vi "Parameter.vi"(9 "In":string, 10 "VIId":string, 11 "VariablesRef":T4) -> ()   [LabVIEW 2018, in "TDKDCSource.lvlib"]
uses:
  TDKDCSource.lvlib
  <userlib>/_OpenG.lib/dictionary/dictionary.llb/Dictionary Object RefNum__ogtk.ctl
  <userlib>/_OpenG.lib/dictionary/dictionary.llb/Dictionary Object RefNum - Enum__ogtk.ctl
  <vilib>/addons/_JKI.lib/Serialization/JSON/JKI JSON Serialization.lvlib
panel:
  in  "Tab Control":enum32{"Config", "控件"}(tab)
  in  "ArrayType":T1(tab)
  in  "Configuration":T2={"Language Selector"=enum."SCPI", "Baud Rate"=enum."9600", "Address"=6}
  in  "TDK直流电源端口":refnum<visa-resource-name>
  in  "Reset Device":bool
  in  "ID Query":bool
  in  "方法(Method)":T3(ring)
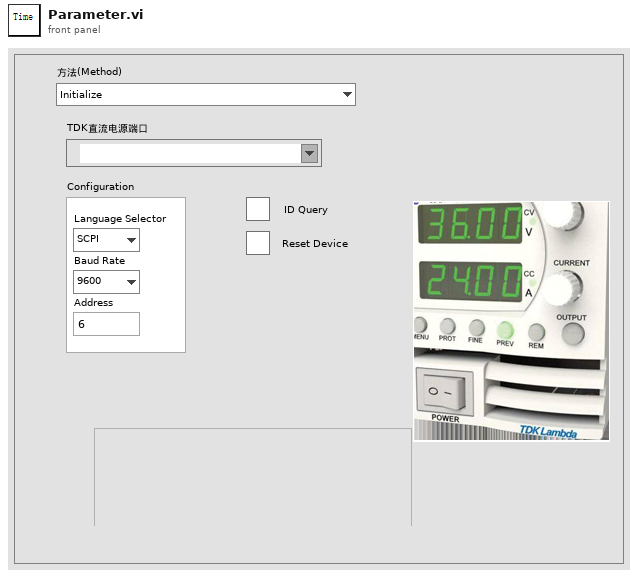
[diagram p1: front panel]
types:
  T1 = enum32{"Initialize", "SetVoltage", "SetCurrent", "SetOutput", "SetProtectedVoltage", "GetCurrent", "GetVoltage"}
  T2 = cluster{"Language Selector":enum16{"GEN", "SCPI"}, "Baud Rate":enum16{"1200", "2400", "4800", "9600", "19200", "38400", "57600", "115200"}, "Address":i16}
  T3 = enum16{"Initialize", "SetVoltage", "SetCurrent", "SetOutput", "SetProtectedVoltage", "GetCurrent", "GetVoltage", "GetPower"}
  T4 = typedef "Dictionary Object RefNum__ogtk.ctl" = refnum<k1>
  T5 = cluster{"Initialize":cluster{"json":cluster{"Method":string, "Time":i32, "ID Query":bool, "Reset Device":bool}}, "SetVoltage":cluster{"json":cluster{"Method":string, "Time":i32}}, "SetCurrent":cluster{"json":cluster{"Method":string}}}
  T6 = enum32{"Invalid", "Standard", "Closed", "Hidden", "Minimized", "Maximized"}
  T7 = enum32{"invalid app kind", "Development System", "Run Time System", "Student Edition", "Embedded LabVIEW", "Evaluation", "Custom"}
  T8 = cluster{"Core":cluster{"Current VI Reference":refnum<vi>, "Close Panel on Exit?":bool}, "Parameter":cluster{"VariableRef":T4}, "Synchronize":cluster{"EnqueueData":cluster{"Action":enum16{"Create", "Query", "Revert", "UpdateVariable", "Close"}, "Data":variant}, "Echo":cluster{"VIRef":refnum<vi>, "JsonOut":string, "Status":string}, "Communicate":cluster{"ID":string, "JsonIn":string, "VarRef":T4}, "Queue":refnum<queue>}, "TimeClusters":cluster{"Initialize":cluster{"json":cluster{"Method":string, "Time":i32, "ID Query":bool, "Reset Device":bool}}, "SetVoltage":cluster{"json":cluster{"Method":string, "Time":i32}}, "SetCurrent":cluster{"json":cluster{"Method":string}}}}
  T9 = cluster{"EnqueueData":cluster{"Action":enum16{"Create", "Query", "Revert", "UpdateVariable", "Close"}, "Data":variant}, "Echo":cluster{"VIRef":refnum<vi>, "JsonOut":string, "Status":string}, "Communicate":cluster{"ID":string, "JsonIn":string, "VarRef":T4}, "Queue":refnum<queue>}
  T10 = cluster{"Current VI Reference":refnum<vi>, "Close Panel on Exit?":bool}
  T11 = cluster{"json":cluster{"Method":string, "Time":i32, "ID Query":bool, "Reset Device":bool}}
  T12 = cluster{"json":cluster{"Method":string, "Time":i32}}
  T13 = cluster{"Action":enum16{"Create", "Query", "Revert", "UpdateVariable", "Close"}, "Data":variant}
  T14 = cluster{"ID":string, "JsonIn":string, "VarRef":T4}
  T15 = enum16{"Create", "Query", "Revert", "UpdateVariable", "Close"}
  T16 = cluster{"VIRef":refnum<vi>, "JsonOut":string, "Status":string}
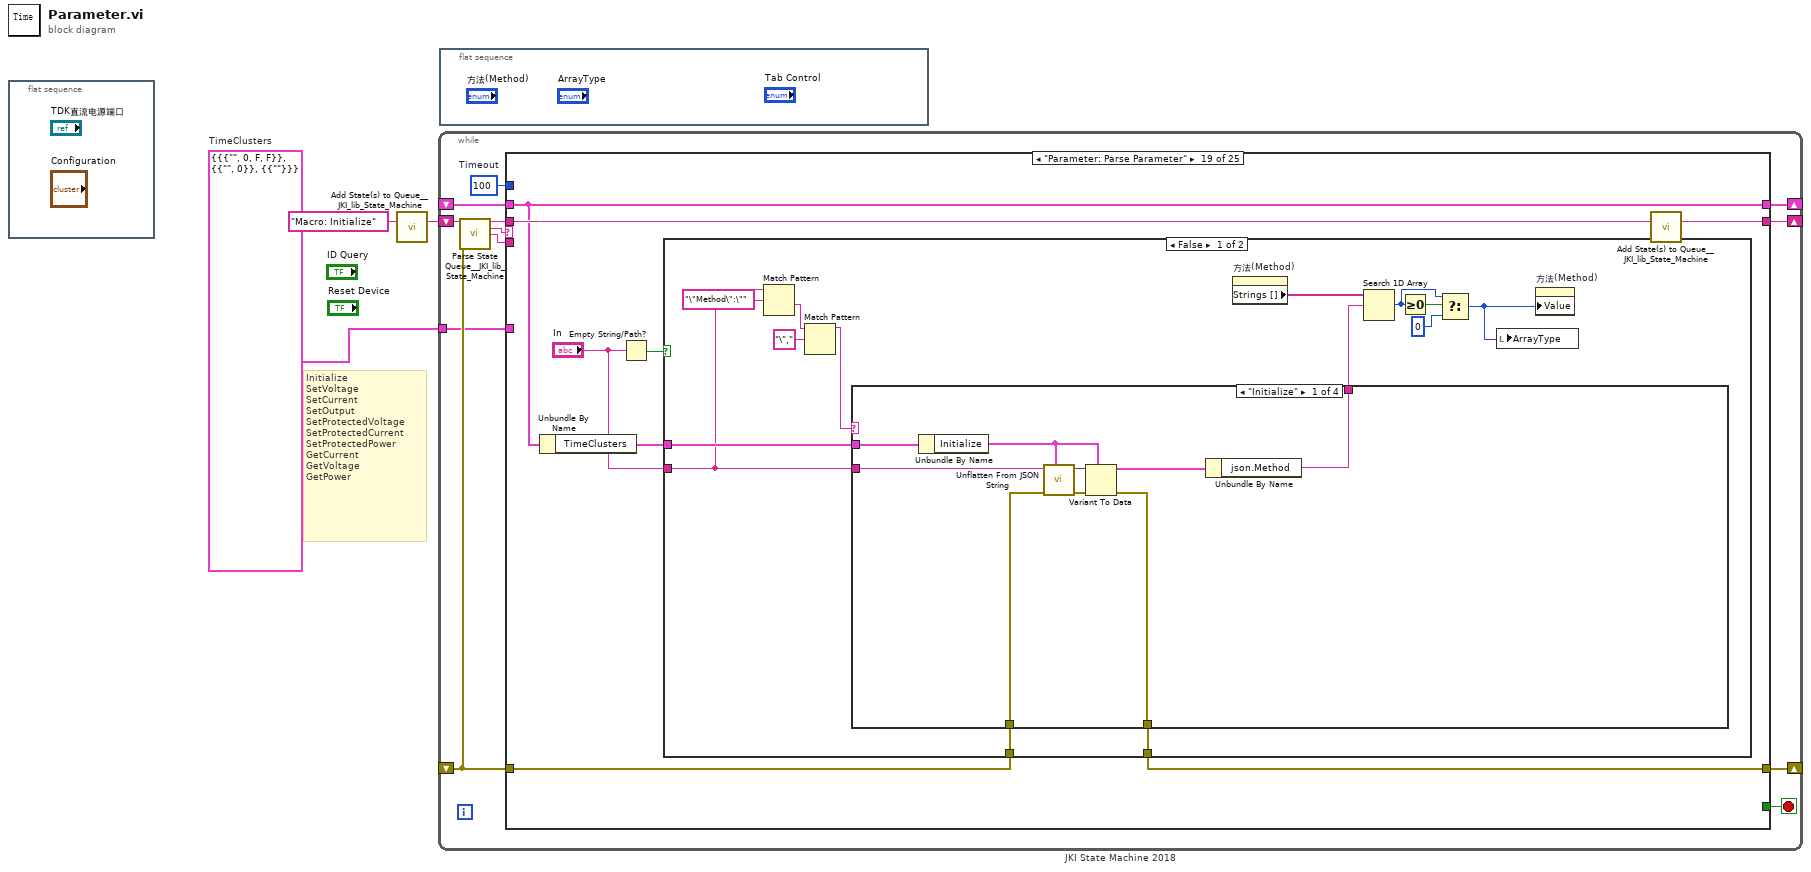
[diagram p0: block diagram]
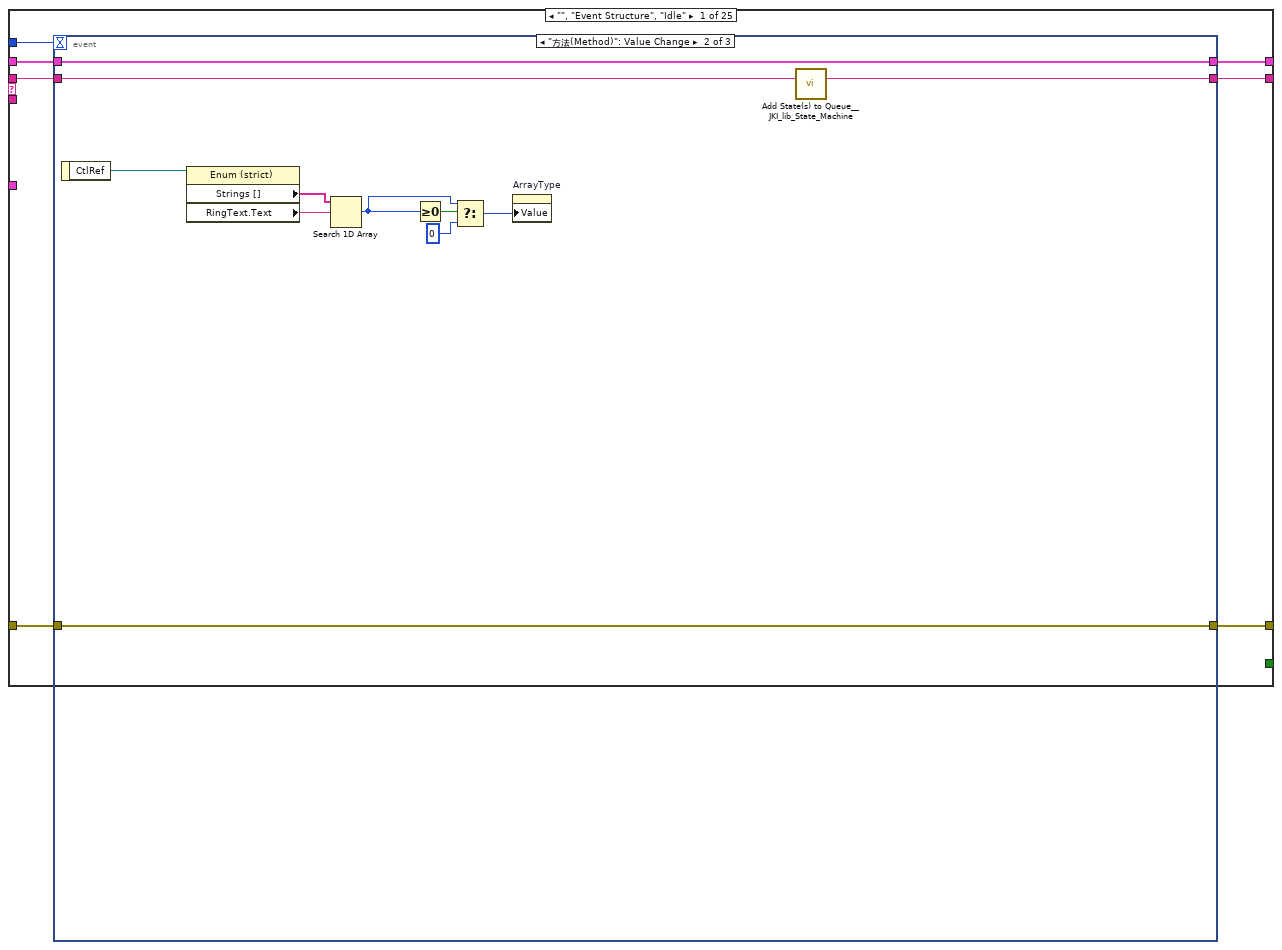
[diagram p2: hidden frame]
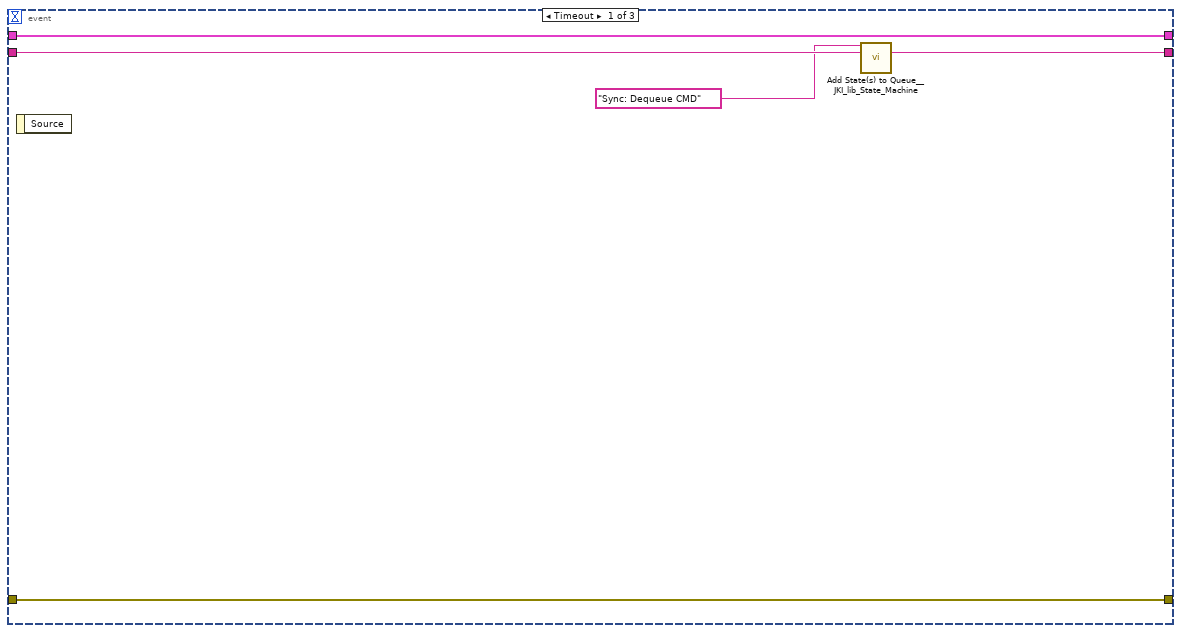
[diagram p3: hidden frame]
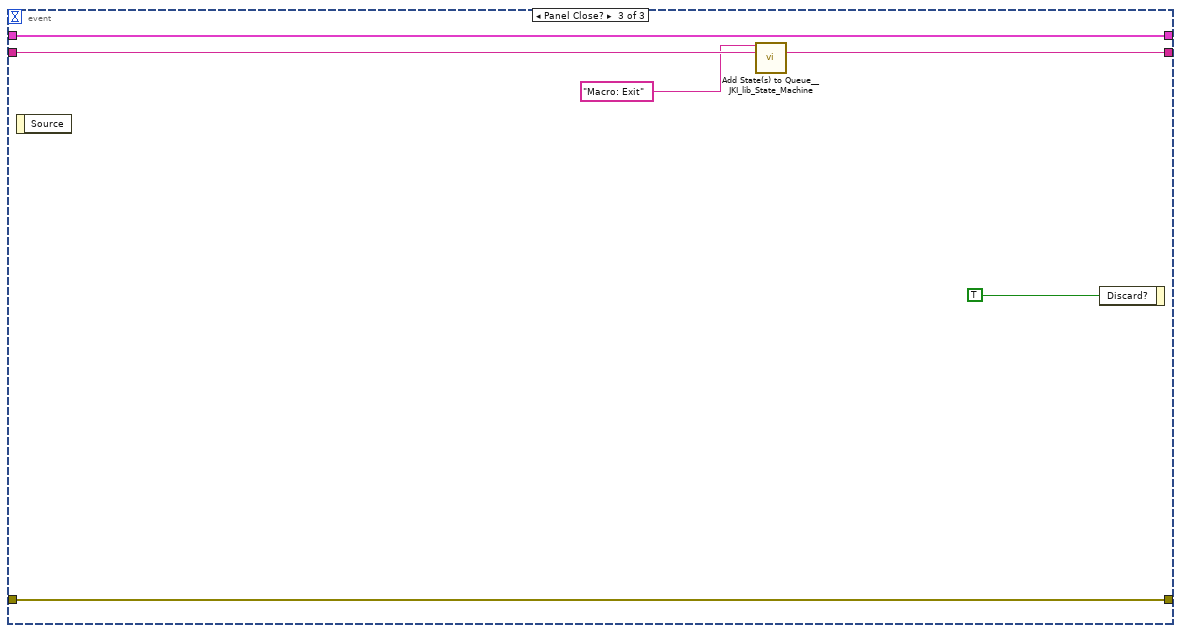
[diagram p4: hidden frame]
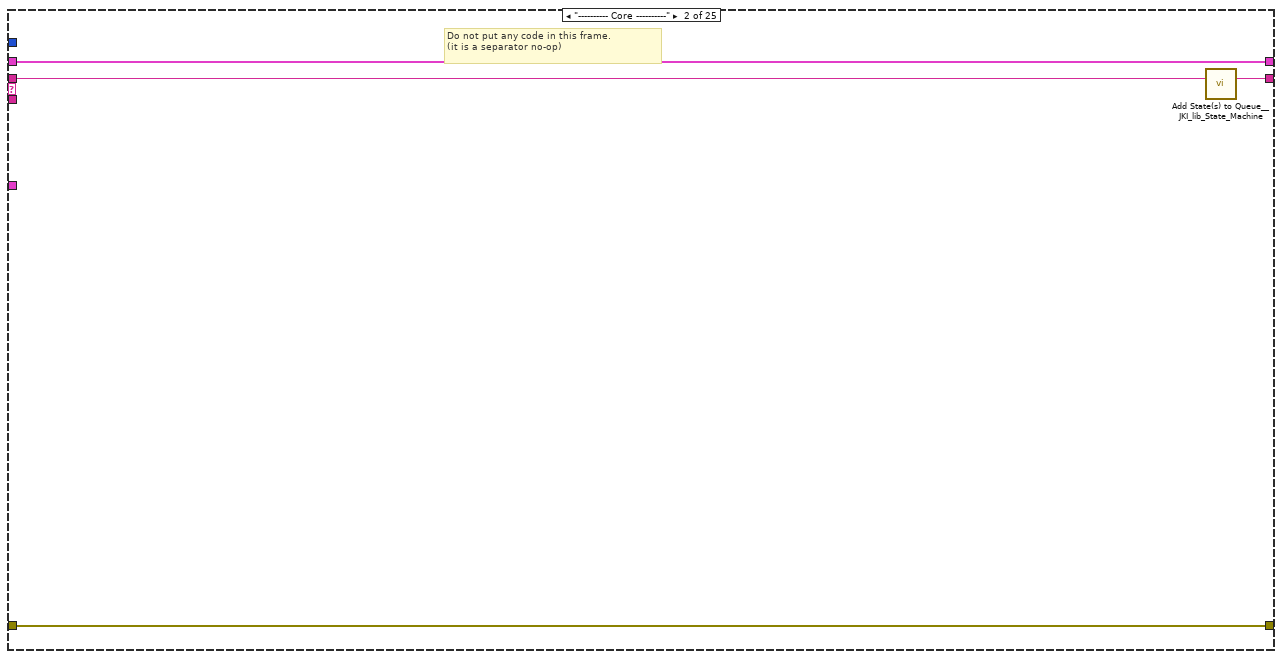
[diagram p5: hidden frame]
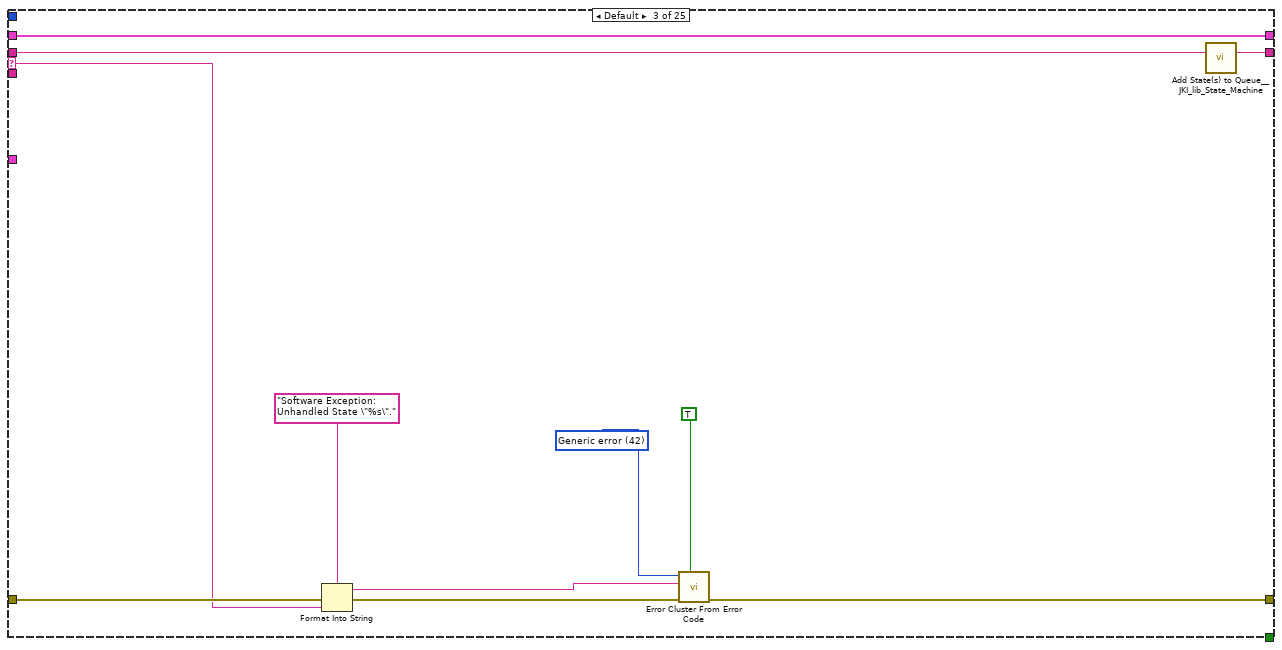
[diagram p6: hidden frame]
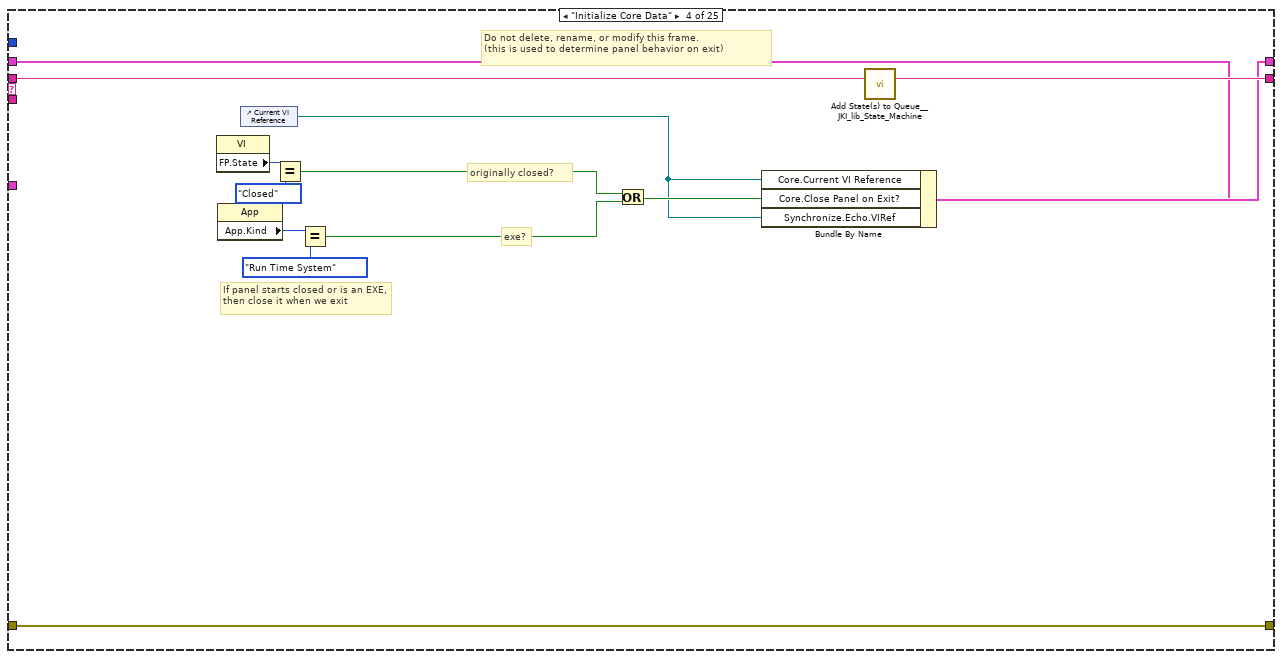
[diagram p7: hidden frame]
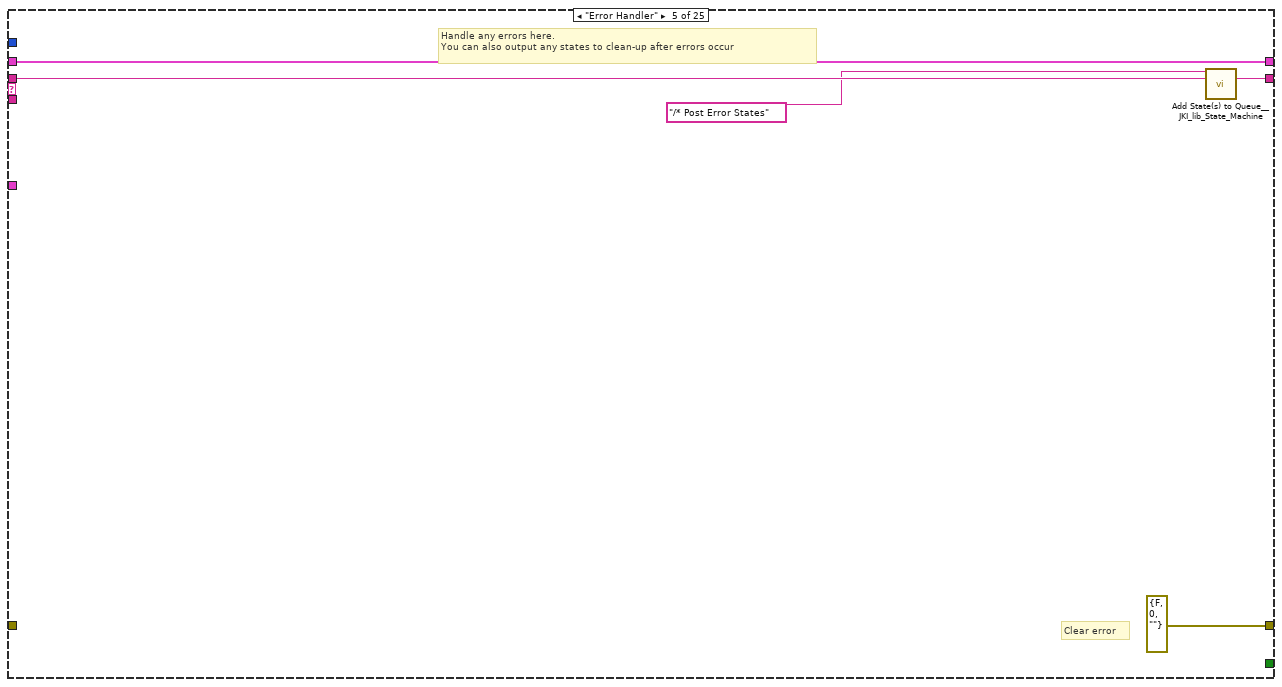
[diagram p8: hidden frame]
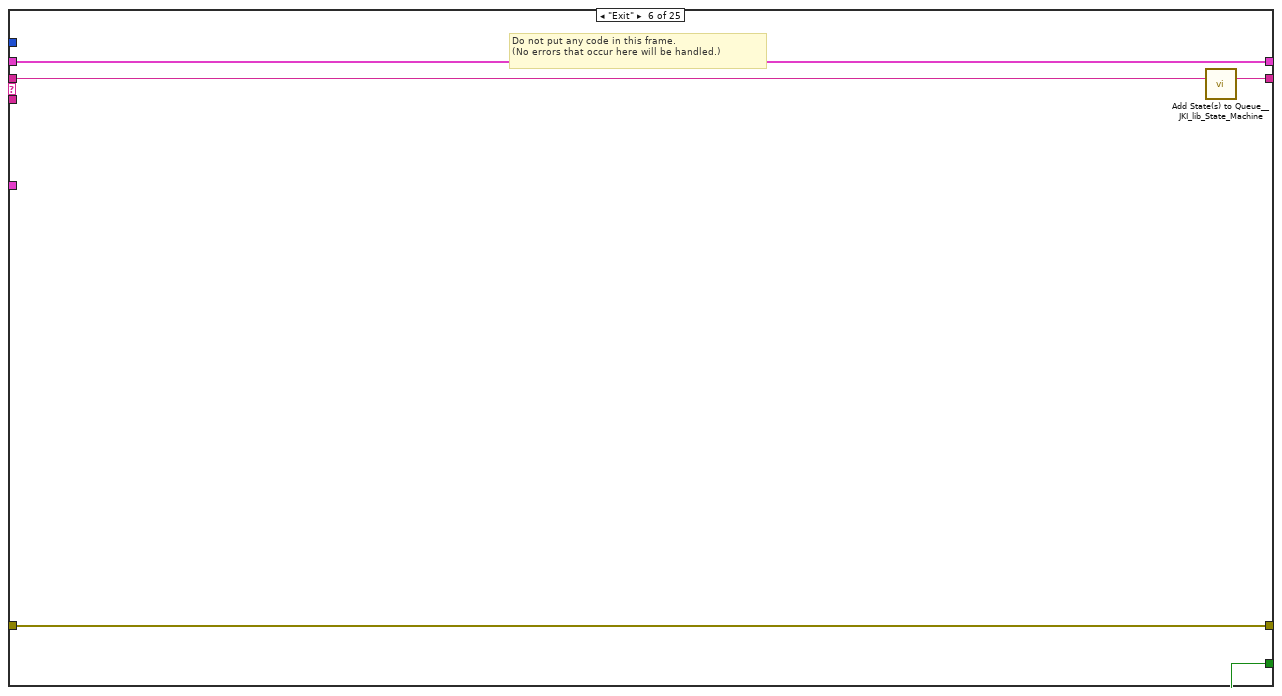
[diagram p9: hidden frame]
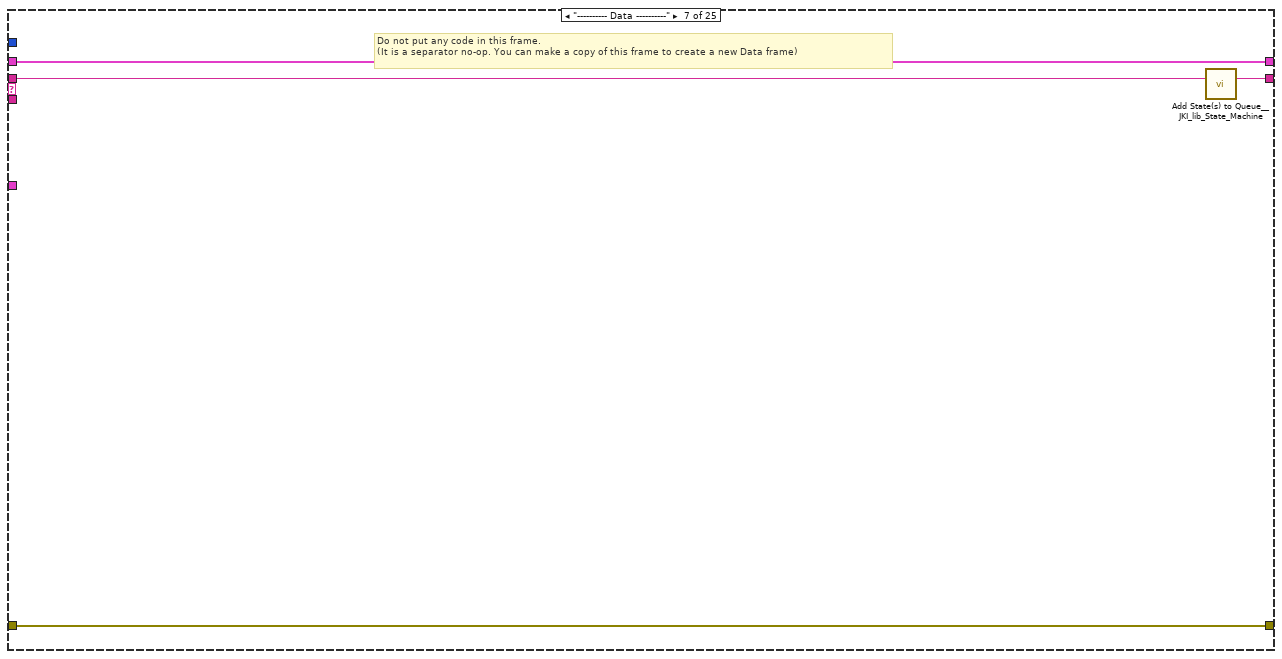
[diagram p10: hidden frame]
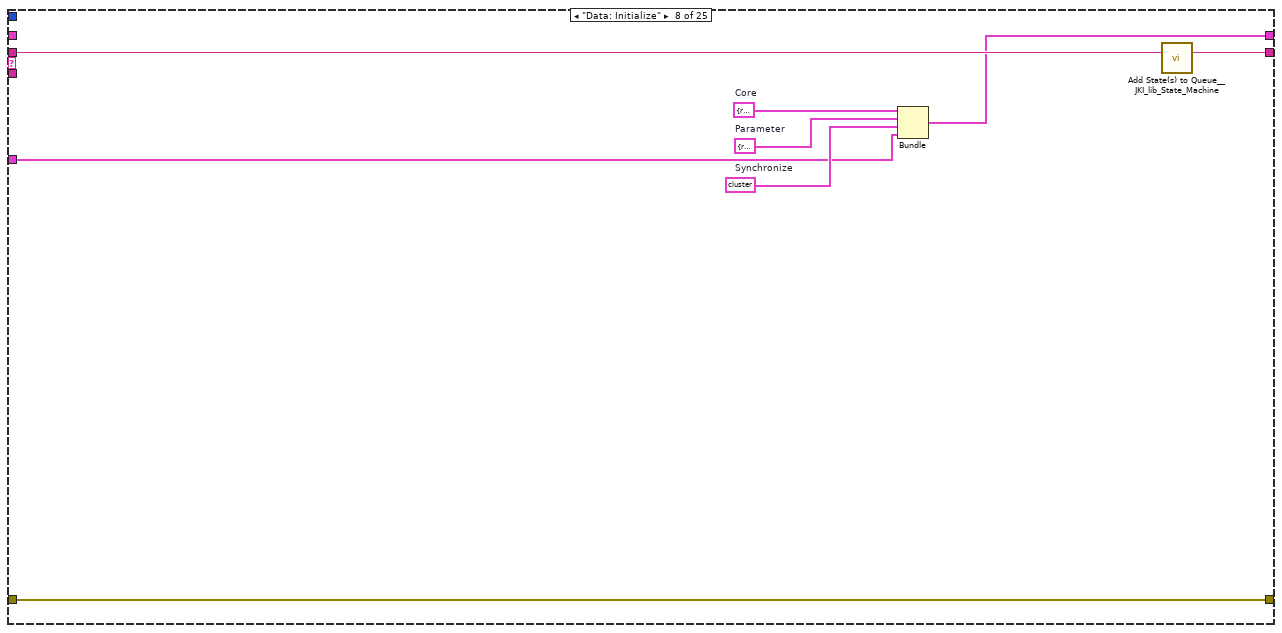
[diagram p11: hidden frame]
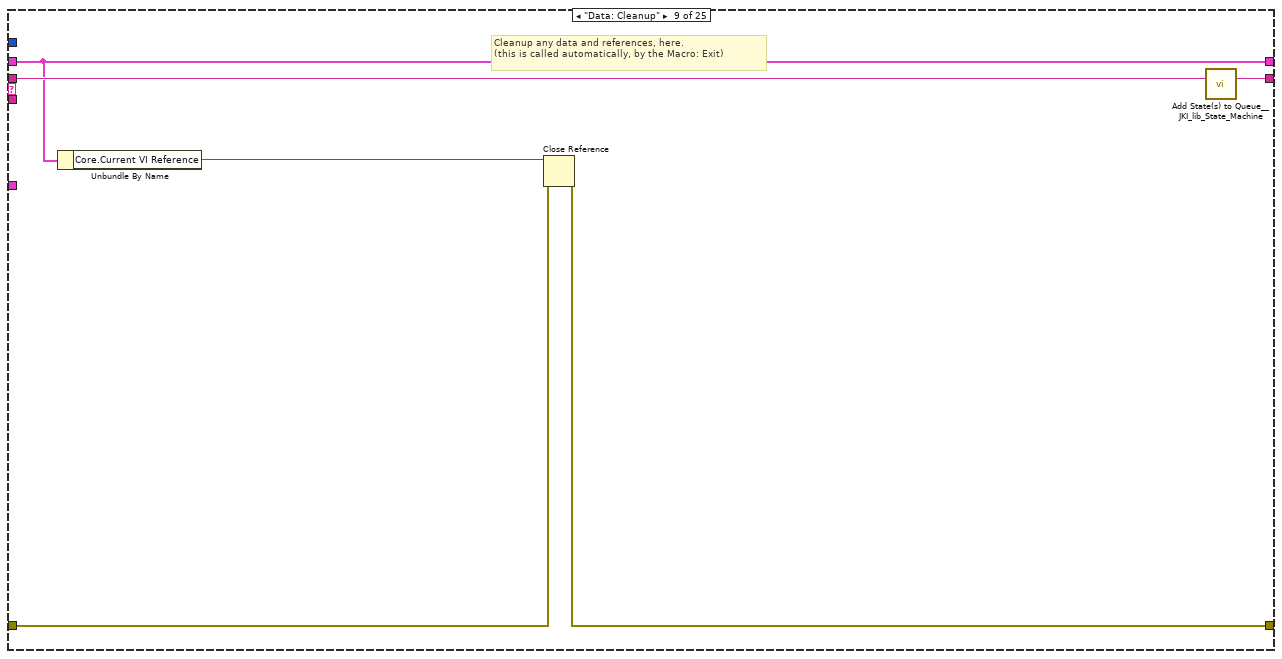
[diagram p12: hidden frame]
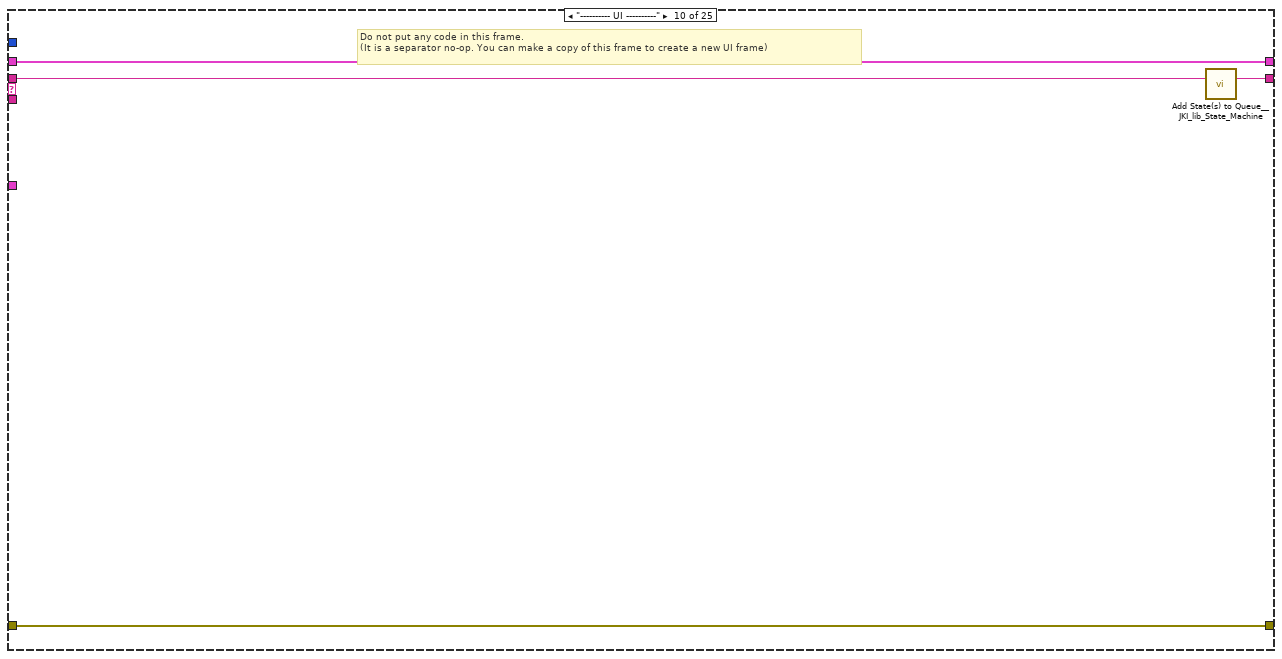
[diagram p13: hidden frame]
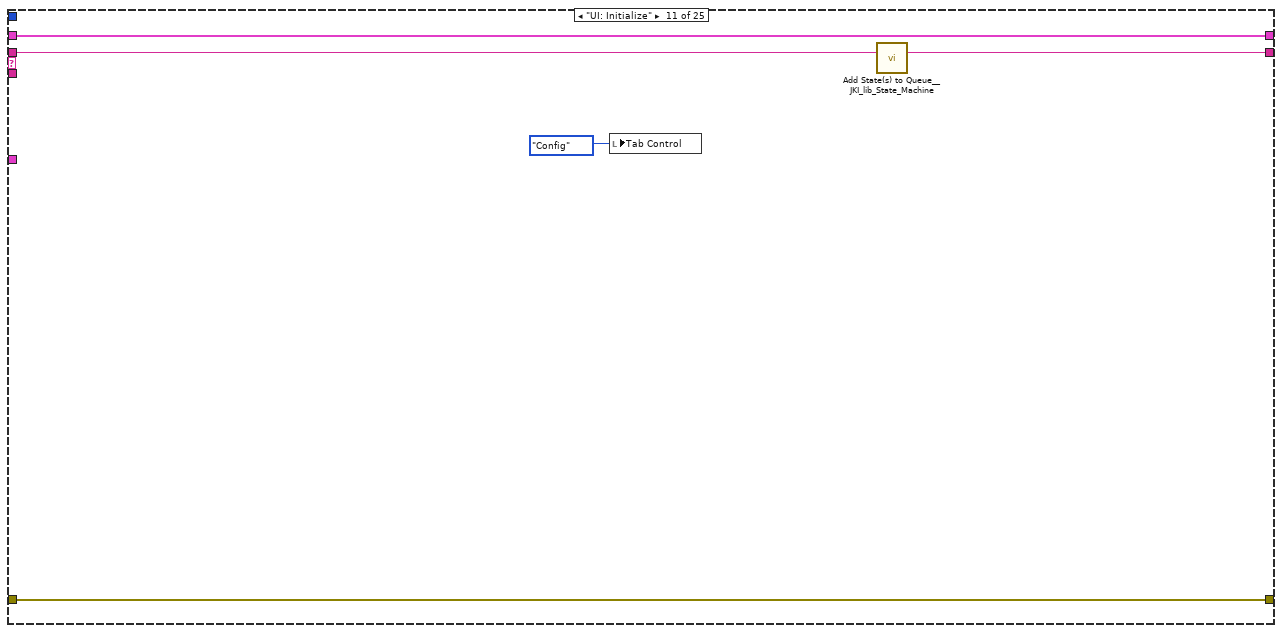
[diagram p14: hidden frame]
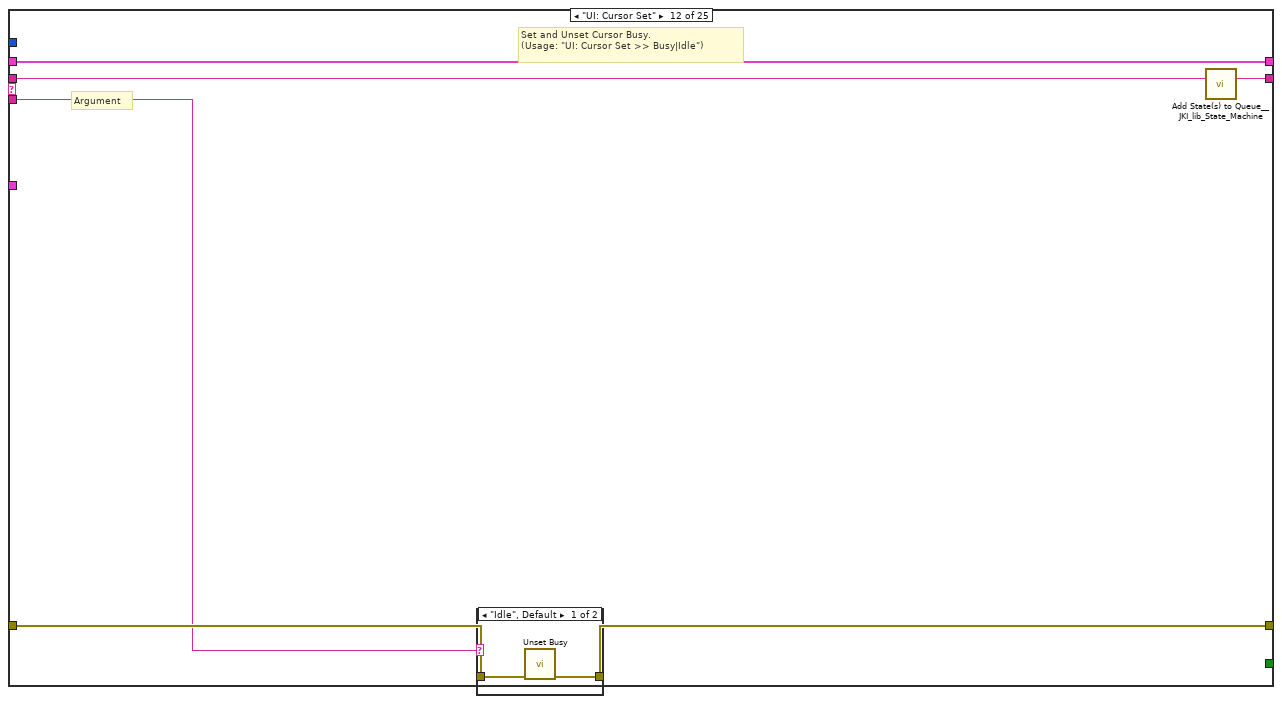
[diagram p15: hidden frame]
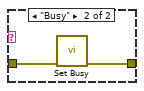
[diagram p16: hidden frame]
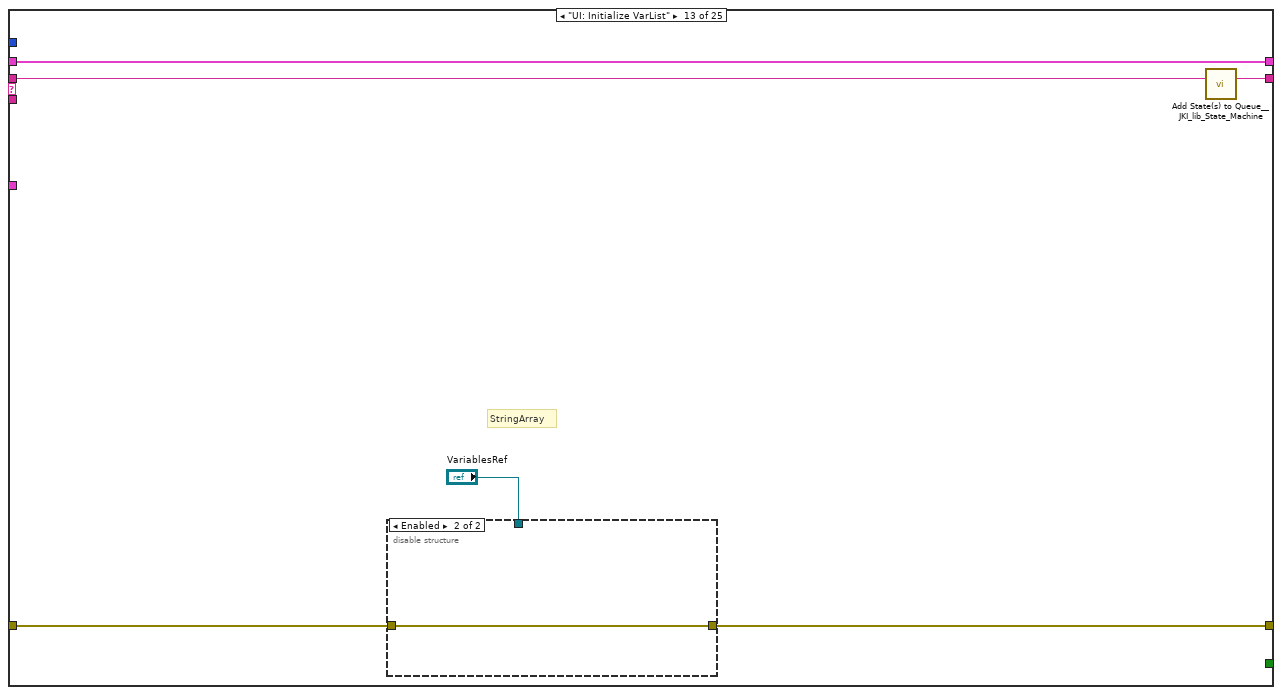
[diagram p17: hidden frame]
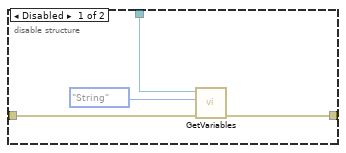
[diagram p18: hidden frame]
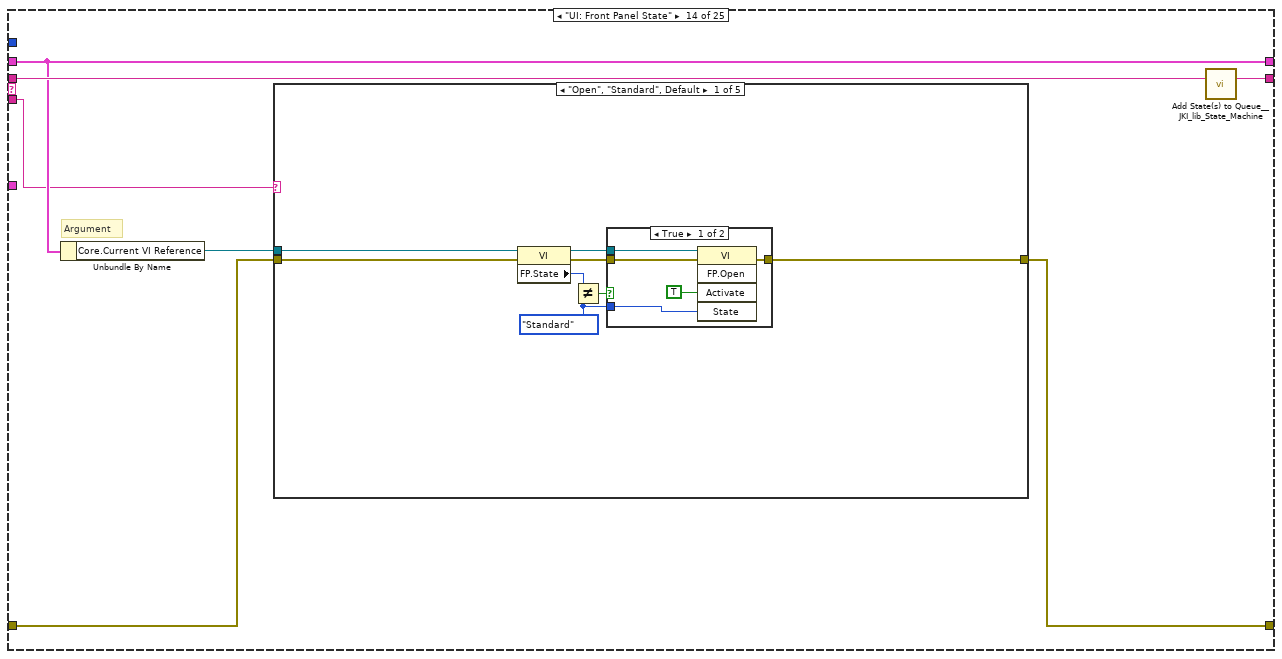
[diagram p19: hidden frame]
diagram:
  w1 = T5 {"Initialize"={"json"={"Method"="", "Time"=0, "ID Query"=FALSE, "Reset Device"=FALSE}}, "SetVoltage"={"json"={"Method"="", "Time"=0}}, "SetCurrent"={"json"={"Method"=""}}}  # TimeClusters
  # "Initialize\nSetVoltage\nSetCurrent\nSetOutput\nSetProtectedVoltage\nSetProtectedCurrent\nSetProtectedPower\nGetCurrent\nGetVoltage\nGetPower"
  n1 = flat-sequence {
    frame #0 {
    }
  }
  n2 = call <vilib>:"Add State(s) to Queue__JKI_lib_State_Machine.vi"("State(s) in (\"\")"="Macro: Initialize") -> ("States Out"=w3:string)  [unwired: 14 in]
  n3 = while "JKI State Machine 2018" {
    shift-right: [w8] -> _
    shift-left: _ -> [w7]
    shift-right: [w11] -> _
    shift-left: _ -> [w5]
    shift-right: [w10] -> _
    shift-left: w3 -> [w12]
    tunnel: w1 -> [w4]
    stop <- w9 stop-if-true
    w6 = 100  # Timeout
    n4 = call <vilib>:"Parse State Queue__JKI_lib_State_Machine.vi"("State Queue"=w12, "Error In (no error)"=w5) -> ("Remaining States"=w14:string, "Current State"=w15:string, "Arguments"=w13:string)  [unwired: 11 in]
    n5 = case shown="\"Parameter: Parse Parameter\"" w15 {
      selector: w15 -> [_ _ w49 _ _ _ _ _ _ _ _ _ _ _ _ _ _ _ _ _ _ _ _ _ _]
      tunnel: w14 -> [w22 w48 w53 w72 w77 w82 w86 w94 w100 w104 w109 w115 w125 w137 w206 w211 w221 w225 w233 w285 w314 w323 w338 w382 w397]
      tunnel: w13 -> [_ _ _ _ _ _ _ _ _ _ _ w110 _ w131 _ _ _ _ _ _ _ _ _ _ _]
      tunnel: w7 -> [w20 w45 w51 w65 w74 w80 w83 _ w95 w101 w106 w113 w123 w133 w203 w208 w218 w222 w228 w278 w311 w316 w336 w379 w386]
      tunnel: [w19 w46 w55 w69 errorcluster {"status"=FALSE, "code"=0, "source"=""} ("error out") w79 w84 w92 w96 w102 w105 w111 w120 w134 w204 w209 w219 w223 w229 w282 w312 w320 w325 w377 w384] -> w11
      tunnel: w5 -> [w18 w46 w54 w69 _ w79 w84 w92 w97 w102 w105 w112 w121 w135 w204 w209 w219 w223 w230 w281 w312 w321 w334 w378 w385]
      tunnel: [w21 w47 w52 w71 w76 w81 w85 w93 w99 w103 w108 w114 w124 w136 w205 w210 w220 w224 w232 w284 w313 w322 w337 w381 w396] -> w10
      tunnel: [_ _ _ _ _ TRUE _ _ _ _ _ _ _ _ _ _ _ _ _ _ _ _ _ _ _] -> w9
      tunnel: [w17 w45 w51 w70 w74 w80 w83 w89 w95 w101 w106 w113 w123 w133 w203 w208 w218 w222 w228 w283 w311 w318 w327 w379 w386] -> w8
      tunnel: w6 -> [w16 _ _ _ _ _ _ _ _ _ _ _ _ _ _ _ _ _ _ _ _ _ _ _ _]
      tunnel: w4 -> [_ _ _ _ _ _ _ w87 _ _ _ _ _ _ _ _ _ _ _ _ _ _ _ _ _]
      frame "", "Event Structure", "Idle" {
        n6 = event shown="[1] \"方法(Method)\": Value Change" {
          selector: _ -> [_ _ _]
          dyn-events: _ -> [_ _ _]
          timeout: w16 -> [_ _ _]
          tunnel: w22 -> [w27 w38 w44]
          tunnel: [w26 w37 w43] -> w21
          tunnel: w20 -> [w24 w35 w41]
          tunnel: [w25 w36 w42] -> w19
          tunnel: w18 -> [w25 w36 w42]
          tunnel: [w24 w35 w41] -> w17
          event Timeout {
            n7 = event-data() -> ()  [unwired: 1 in, 1 out]
            n8 = call <vilib>:"Add State(s) to Queue__JKI_lib_State_Machine.vi"("State(s) in Front (\"\")"="Sync: Dequeue CMD" ("State(s) in Front (\"\")"), "State(s) in (\"\")"=w27) -> ("States Out"=w26:string)  [unwired: 13 in]
          }
          event "方法(Method)": Value Change {
            n9 = event-data() -> ("CtlRef"=w31:refnum<vi>)  [unwired: 1 in]
            n10 = property class="Enum (strict)"(reference=w31) -> ("Strings []"=w30:string[], "RingText.Text"=w29:string)  [unwired: 1 in, 2 out]
            n11 = Search 1D Array(1D array=w30, element=w29) -> (index of element=w33:i32)  [unwired: 1 in]
            n12 = Greater Or Equal To 0?(x=w33) -> (x >= 0?=w34:bool)
            n13 = Select(t=w33, s=w34, f=0) -> (s? t:f=w28:i32)
            n14 = property on="ArrayType" class="TabCtl (strict)"("Value"=w28) -> ()  [unwired: 2 in, 2 out]
            n15 = call <vilib>:"Add State(s) to Queue__JKI_lib_State_Machine.vi"("State(s) in (\"\")"=w38) -> ("States Out"=w37:string)  [unwired: 14 in]
          }
          event Panel Close? {
            n16 = event-data() -> ()  [unwired: 1 in, 1 out]
            n17 = call <vilib>:"Add State(s) to Queue__JKI_lib_State_Machine.vi"("State(s) in Front (\"\")"="Macro: Exit", "State(s) in (\"\")"=w44) -> ("States Out"=w43:string)  [unwired: 13 in]
            n18 = event-data("Discard?"=TRUE) -> ()  [unwired: 1 in, 1 out]
          }
        }
      }
      frame "---------- Core ----------" {
        # "Do not put any code in this frame.\n(it is a separator no-op)"
        n19 = call <vilib>:"Add State(s) to Queue__JKI_lib_State_Machine.vi"("State(s) in (\"\")"=w48) -> ("States Out"=w47:string)  [unwired: 14 in]
      }
      frame Default {
        w58 = 42 items=["No error", "Argument error", "Memory is full", "Out of zone", "End of file", "File already open", "Generic file I/O error", "File not found", "File permission error", "Disk is full", "Duplicate path", "Too many files open", "System feature not enabled", "Resource file not found", "Cannot add resource", "Resource not found", "Image not found", "Image memory error", "Pen does not exist", "Config type invalid", "Config token not found", "Config parse error", "Config memory error", "Bad external code format", "Bad external code offset", "External code not present", "Null window", "Destroy window error", "Null menu", "Print aborted", "Bad print record", "Print driver error", "Windows error during printing", "Memory error during printing", "Print dialog error", "Generic print error", "Invalid device refnum", "Device not found", "Device parameter error", "Device unit error", "Cannot open device", "Device call aborted", "Generic error", "Cancelled by user", "Object ID too low", "Object ID too high", "Object not in heap", "Unknown heap", "Unknown object (invalid DefProc)", "Unknown object (DefProc not in table)", "Message out of range", "Invalid (null) method", "Unknown message", "Manager call not supported", "Bad address", "Network operation in progress", "Network operation timed out", "Connection is busy", "Network attribute not supported", "Network error", "Address in use", "System out of memory", "Connection aborted", "Connection refused", "Not connected", "Already connected", "Connection closed", "Initialization error (interapplication manager)", "Bad occurrence", "Wait on unbound occurrence handler", "Occurrence queue overflow", "Datalog type conflict", "Unused", "Unrecognized type (interapplication manager)", "Memory corrupt", "Failed to make temporary DLL", "Old CIN version", "Drag socket not found", "Failed to load drop-object", "Failed to register OLE object", "Failed to release OLE object", "Format specifier type mismatch", "Unknown format specifier", "Too few format specifiers", "Too many format specifiers", "Scan failed", "Newer CIN version", "Error converting to variant", "Runtime menu error", "Password tampered", "Variant attribute not found", "Incompatible variant data type", "Event data is not available", "Event Store is not present", "Occurrence is not found", "Event Queue is not created", "Event info is not available", "Refnum passed is NULL", "Error retrieving Class GUID", "Error retrieving CoClass GUID", "Error retrieving TypeLib GUID.", "Bad built application magic bytes.", "Specific driver is different from the specific driver associated with the Logical Name.", "There is no session opened to the class driver.", "Max Error", "MAX - Error with config objects", "MAX - Error loading configuration", "MAX - Group not supported"]
        n20 = Format Into String(format string="Software Exception: Unhandled State \"%s\"." ("message"), error in=w54, w49) -> (resulting string=w57:string, error out=w56:errorcluster)  [unwired: 1 in]
        n21 = call <vilib>:"Error Cluster From Error Code.vi"("show call chain? (False)"=TRUE, "error in (no error)"=w56, "error message (\"\")"=w57, "error code (0)"=w58) -> ("error out"=w55:errorcluster)  [unwired: 5 in]
        n22 = call <vilib>:"Add State(s) to Queue__JKI_lib_State_Machine.vi"("State(s) in (\"\")"=w53) -> ("States Out"=w52:string)  [unwired: 14 in]
      }
      frame "Initialize Core Data" {
        # "Do not delete, rename, or modify this frame.\n(this is used to determine panel behavior on exit)"
        # "originally closed?"
        # "exe?"
        # "If panel starts closed or is an EXE, then close it when we exit"
        n23 = property class="VI"() -> ("FP.State"=w63:T6)  [unwired: 2 in, 2 out]
        n24 = property class="App"() -> ("App.Kind"=w68:T7)  [unwired: 2 in, 2 out]
        n25 = control-ref of="Current VI Reference"() -> (w60:refnum<vi>)
        n26 = Equal?(x=w63, y=T6."Closed" ("Front Panel Window:State")) -> (x = y?=w61:bool)
        n27 = Equal?(x=w68, y=T7."Run Time System" ("Application:Kind")) -> (x = y?=w66:bool)
        n28 = Or(x=w61, y=w66) -> (x .or. y?=w64:bool)
        n29 = Bundle By Name(cluster=w65, "Core.Current VI Reference"=w60, "Core.Close Panel on Exit?"=w64, "Synchronize.Echo.VIRef"=w60) -> (w70:T8)
        n30 = call <vilib>:"Add State(s) to Queue__JKI_lib_State_Machine.vi"("State(s) in (\"\")"=w72) -> ("States Out"=w71:string)  [unwired: 14 in]
      }
      frame "Error Handler" {
        # "Handle any errors here.\nYou can also output any states to clean-up after errors occur"
        # "Clear error"
        n31 = call <vilib>:"Add State(s) to Queue__JKI_lib_State_Machine.vi"("State(s) in Front (\"\")"="/* Post Error States", "State(s) in (\"\")"=w77) -> ("States Out"=w76:string)  [unwired: 13 in]
      }
      frame "Exit" {
        # "Do not put any code in this frame.\n(No errors that occur here will be handled.)"
        n32 = call <vilib>:"Add State(s) to Queue__JKI_lib_State_Machine.vi"("State(s) in (\"\")"=w82) -> ("States Out"=w81:string)  [unwired: 14 in]
      }
      frame "---------- Data ----------" {
        # "Do not put any code in this frame.\n(It is a separator no-op. You can make a copy of this frame to create a new Data frame)"
        n33 = call <vilib>:"Add State(s) to Queue__JKI_lib_State_Machine.vi"("State(s) in (\"\")"=w86) -> ("States Out"=w85:string)  [unwired: 14 in]
      }
      frame "Data: Initialize" {
        w88 = cluster{"VariableRef":T4} {"VariableRef"=refnum}  # Parameter
        w90 = T9 {"EnqueueData"={"Action"=enum."Create", "Data"=variant}, "Echo"={"VIRef"=refnum, "JsonOut"="", "Status"=""}, "Communicate"={"ID"="", "JsonIn"="", "VarRef"=refnum}, "Queue"=refnum}  # Synchronize
        w91 = T10 {"Current VI Reference"=refnum, "Close Panel on Exit?"=FALSE}  # Core
        n34 = Bundle("Core"=w91, "Parameter"=w88, "Synchronize"=w90, "TimeClusters"=w87) -> (w89:T8)  [unwired: 1 in]
        n35 = call <vilib>:"Add State(s) to Queue__JKI_lib_State_Machine.vi"("State(s) in (\"\")"=w94) -> ("States Out"=w93:string)  [unwired: 14 in]
      }
      frame "Data: Cleanup" {
        # "Cleanup any data and references, here.\n(this is called automatically, by the Macro: Exit)"
        n36 = Unbundle By Name(w95) -> ("Core.Current VI Reference"=w98:refnum<vi>)
        n37 = Close Reference(reference=w98, error in (no error)=w97) -> (error out=w96:errorcluster)
        n38 = call <vilib>:"Add State(s) to Queue__JKI_lib_State_Machine.vi"("State(s) in (\"\")"=w100) -> ("States Out"=w99:string)  [unwired: 14 in]
      }
      frame "---------- UI ----------" {
        # "Do not put any code in this frame.\n(It is a separator no-op. You can make a copy of this frame to create a new UI frame)"
        n39 = call <vilib>:"Add State(s) to Queue__JKI_lib_State_Machine.vi"("State(s) in (\"\")"=w104) -> ("States Out"=w103:string)  [unwired: 14 in]
      }
      frame "UI: Initialize" {
        n40 = local write "Tab Control"(enum32{"Config", "控件"}."Config" ("Tab Control")) -> ()
        n41 = call <vilib>:"Add State(s) to Queue__JKI_lib_State_Machine.vi"("State(s) in (\"\")"=w109) -> ("States Out"=w108:string)  [unwired: 14 in]
      }
      frame "UI: Cursor Set" {
        # "Argument"
        # "Set and Unset Cursor Busy.\n(Usage: \"UI: Cursor Set >> Busy|Idle\")"
        n42 = case shown="\"Idle\", Default" w110 {
          tunnel: w112 -> [w117 w119]
          tunnel: [w116 w118] -> w111
          frame "Idle", Default {
            n43 = call <vilib>:"Unset Busy.vi"("error in (no error)"=w117) -> ("error out"=w116:errorcluster)  [unwired: 10 in]
          }
          frame "Busy" {
            n44 = call <vilib>:"Set Busy.vi"("error in (no error)"=w119) -> ("error out"=w118:errorcluster)  [unwired: 9 in, 1 out]
          }
        }
        n45 = call <vilib>:"Add State(s) to Queue__JKI_lib_State_Machine.vi"("State(s) in (\"\")"=w115) -> ("States Out"=w114:string)  [unwired: 14 in]
      }
      frame "UI: Initialize VarList" {
        # "StringArray"
        n46 = disable-structure shown="Enabled" {
          disable-tunnel: "VariablesRef" -> [w129 _]
          disable-tunnel: w121 -> [w127 w130]
          disable-tunnel: [w126 w130] -> w120
          frame Disabled {
            n47 = call "GetVariables.vi"("error in (no error)"=w127, "VariableType"=enum16{"String", "StringArray"}."String", "DicRef"=w129) -> ("error out"=w126:errorcluster)  [unwired: 7 in, 1 out]
          }
          frame Enabled {
          }
        }
        n48 = call <vilib>:"Add State(s) to Queue__JKI_lib_State_Machine.vi"("State(s) in (\"\")"=w125) -> ("States Out"=w124:string)  [unwired: 14 in]
      }
      frame "UI: Front Panel State" {
        # "Argument"
        n49 = Unbundle By Name(w133) -> ("Core.Current VI Reference"=w132:refnum<vi>)
        n50 = case shown="\"Open\", \"Standard\", Default" w131 {
          tunnel: w135 -> [w143 w158 w169 w182 w195]
          tunnel: [w145 w159 w171 w184 w197] -> w134
          tunnel: w132 -> [w144 w156 w170 w183 w196]
          frame "Open", "Standard", Default {
            w138 = T6."Standard" ("State")
            n51 = property class="VI"(reference=w144, error in=w143) -> (reference out=w141:refnum<vi>, error out=w142:errorcluster, "FP.State"=w140:T6)
            n52 = Not Equal?(x=w140, y=w138) -> (x != y?=w139:bool)
            n53 = case shown="True" w139 {
              tunnel: [w149 w151] -> w145
              tunnel: w142 -> [w148 w151]
              tunnel: w141 -> [w147 _]
              tunnel: w138 -> [w146 _]
              frame True {
                n54 = invoke class="VI" method="FP.Open"(reference=w147, error in=w148, "Activate"=TRUE, "State"=w146) -> (error out=w149:errorcluster)  [unwired: 1 in, 4 out]
              }
              frame False {
              }
            }
          }
          frame "Close", "Closed" {
            n55 = property class="VI"(reference=w156, error in=w158) -> (reference out=w155:refnum<vi>, error out=w157:errorcluster, "FP.State"=w153:T6)
            n56 = Not Equal?(x=w153, y=T6."Closed" ("Front Panel Window:State")) -> (x != y?=w152:bool)
            n57 = case shown="True" w152 {
              tunnel: [w160 w163] -> w159
              tunnel: w157 -> [w160 w162]
              tunnel: w155 -> [_ w161]
              frame False {
              }
              frame True {
                n58 = invoke class="VI" method="FP.Close"(reference=w161, error in=w162) -> (error out=w163:errorcluster)  [unwired: 1 in, 2 out]
              }
            }
          }
          frame "Hidden", "Hide" {
            w164 = T6."Hidden" ("State")
            n59 = property class="VI"(reference=w170, error in=w169) -> (reference out=w167:refnum<vi>, error out=w168:errorcluster, "FP.State"=w166:T6)
            n60 = Not Equal?(x=w166, y=w164) -> (x != y?=w165:bool)
            n61 = case shown="True" w165 {
              tunnel: [w175 w176] -> w171
              tunnel: w168 -> [w174 w176]
              tunnel: w167 -> [w173 _]
              tunnel: w164 -> [w172 _]
              frame True {
                n62 = invoke class="VI" method="FP.Open"(reference=w173, error in=w174, "State"=w172) -> (error out=w175:errorcluster)  [unwired: 2 in, 4 out]
              }
              frame False {
              }
            }
          }
          frame "Minimize", "Minimized" {
            w177 = T6."Minimized" ("State")
            n63 = property class="VI"(reference=w183, error in=w182) -> (reference out=w180:refnum<vi>, error out=w181:errorcluster, "FP.State"=w179:T6)
            n64 = Not Equal?(x=w179, y=w177) -> (x != y?=w178:bool)
            n65 = case shown="True" w178 {
              tunnel: [w188 w189] -> w184
              tunnel: w181 -> [w187 w189]
              tunnel: w180 -> [w186 _]
              tunnel: w177 -> [w185 _]
              frame True {
                n66 = invoke class="VI" method="FP.Open"(reference=w186, error in=w187, "State"=w185) -> (error out=w188:errorcluster)  [unwired: 2 in, 4 out]
              }
              frame False {
              }
            }
          }
          frame "Maximize", "Maximized" {
            w190 = T6."Maximized" ("State")
            n67 = property class="VI"(reference=w196, error in=w195) -> (reference out=w193:refnum<vi>, error out=w194:errorcluster, "FP.State"=w192:T6)
            n68 = Not Equal?(x=w192, y=w190) -> (x != y?=w191:bool)
            n69 = case shown="True" w191 {
              tunnel: [w201 w202] -> w197
              tunnel: w194 -> [w200 w202]
              tunnel: w193 -> [w199 _]
              tunnel: w190 -> [w198 _]
              frame True {
                n70 = invoke class="VI" method="FP.Open"(reference=w199, error in=w200, "State"=w198) -> (error out=w201:errorcluster)  [unwired: 2 in, 4 out]
              }
              frame False {
              }
            }
          }
        }
        n71 = call <vilib>:"Add State(s) to Queue__JKI_lib_State_Machine.vi"("State(s) in (\"\")"=w137) -> ("States Out"=w136:string)  [unwired: 14 in]
      }
      frame "---------- Macro ----------" {
        n72 = call <vilib>:"Add State(s) to Queue__JKI_lib_State_Machine.vi"("State(s) in (\"\")"=w206) -> ("States Out"=w205:string)  [unwired: 14 in]
      }
      frame "Macro: Initialize" {
        n73 = call <vilib>:"Add State(s) to Queue__JKI_lib_State_Machine.vi"("State(s) in Front (\"\")"="Data: Initialize\nInitialize Core Data\nUI: Initialize\nSync: Obtain CMD Queue\nSync: Dequeue CMD\nUI: Initialize VarList\nParameter: Parse Parameter", "State(s) in (\"\")"=w211) -> ("States Out"=w210:string)  [unwired: 13 in]
      }
      frame "Macro: Exit" {
        n74 = Unbundle By Name(w218) -> ("Core.Close Panel on Exit?"=w217:bool)
        n75 = Select(t="UI: Front Panel State >> Close", s=w217, f="") -> (s? t:f=w214:string)
        n76 = call <vilib>:"Add State(s) to Queue__JKI_lib_State_Machine.vi"("State(s) in (\"\")"=w214, "State(s) at Back (\"\")"="Sync: Release CMD Queue\nData: Cleanup\nExit") -> ("States Out"=w212:string)  [unwired: 13 in]
        n77 = call <vilib>:"Add State(s) to Queue__JKI_lib_State_Machine.vi"("State(s) in Front (\"\")"=w212, "State(s) in (\"\")"=w221) -> ("States Out"=w220:string)  [unwired: 13 in]
      }
      frame "---------- Parameter ----------" {
        # "Template Separator\n(You can make a copy of, or modify, this frame)"
        n78 = call <vilib>:"Add State(s) to Queue__JKI_lib_State_Machine.vi"("State(s) in (\"\")"=w225) -> ("States Out"=w224:string)  [unwired: 14 in]
      }
      frame "Parameter: Parse Parameter" {
        n79 = Unbundle By Name(w228) -> ("TimeClusters"=w227:T5)
        n80 = Empty String/Path?(string/path="In") -> (empty?=w231:bool)
        n81 = case shown="False" w231 {
          tunnel: "In" -> [w242 _]
          tunnel: w230 -> [w247 w276]
          tunnel: [w246 w276] -> w229
          tunnel: w227 -> [w245 _]
          frame False {
            n82 = Match Pattern(string=w242, regular expression="\"Method\":\"") -> (after substring=w241:string)  [unwired: 1 in, 3 out]
            n83 = Match Pattern(string=w241, regular expression="\",") -> (before substring=w240:string)  [unwired: 1 in, 3 out]
            n84 = case shown="\"Initialize\"" w240 {
              tunnel: w242 -> [w254 w263 w272 _]
              tunnel: w247 -> [w252 w261 w270 w275]
              tunnel: [w251 w260 w269 w275] -> w246
              tunnel: w245 -> [w249 w258 w267 _]
              tunnel: [w250 w259 w268 _] -> w235
              frame "Initialize" {
                n85 = Unbundle By Name(w249) -> ("Initialize"=w248:T11)
                n86 = call <vilib>:"Unflatten From JSON String.vi"("Type and Defaults"=w248, "error in (no error)"=w252, "JSON String"=w254) -> ("error out"=w255:errorcluster, "Variant"=w256:variant)  [unwired: 7 in]
                n87 = Variant To Data(error in=w255, type=w248, Variant=w256) -> (data=w253:T11, error out=w251:errorcluster)
                n88 = Unbundle By Name(w253) -> ("json.Method"=w250:string)
              }
              frame "Wait_s" {
                n89 = Unbundle By Name(w258) -> ("SetVoltage"=w257:T12)
                n90 = call <vilib>:"Unflatten From JSON String.vi"("Type and Defaults"=w257, "error in (no error)"=w261, "JSON String"=w263) -> ("error out"=w264:errorcluster, "Variant"=w265:variant)  [unwired: 7 in]
                n91 = Variant To Data(error in=w264, type=w257, Variant=w265) -> (data=w262:T12, error out=w260:errorcluster)
                n92 = Unbundle By Name(w262) -> ("json.Method"=w259:string)  [unwired: 1 out]
              }
              frame "TickCount" {
                n93 = Unbundle By Name(w267) -> ("SetCurrent"=w266:cluster{"json":cluster{"Method":string}})
                n94 = call <vilib>:"Unflatten From JSON String.vi"("Type and Defaults"=w266, "error in (no error)"=w270, "JSON String"=w272) -> ("error out"=w273:errorcluster, "Variant"=w274:variant)  [unwired: 7 in]
                n95 = Variant To Data(error in=w273, type=w266, Variant=w274) -> (data=w271:cluster{"json":cluster{"Method":string}}, error out=w269:errorcluster)
                n96 = Unbundle By Name(w271) -> ("json.Method"=w268:string)
              }
              frame Default {
              }
            }
            n97 = property on="方法(Method)" class="Enum (strict)"() -> ("Strings []"=w237:string[])  [unwired: 2 in, 2 out]
            n98 = Search 1D Array(1D array=w237, element=w235) -> (index of element=w239:i32)  [unwired: 1 in]
            n99 = Greater Or Equal To 0?(x=w239) -> (x >= 0?=w238:bool)
            n100 = Select(t=w239, s=w238, f=0) -> (s? t:f=w234:i32)
            n101 = local write "ArrayType"(w234) -> ()
            n102 = property on="方法(Method)" class="Enum (strict)"("Value"=w234) -> ()  [unwired: 2 in, 2 out]
          }
          frame True {
          }
        }
        n103 = call <vilib>:"Add State(s) to Queue__JKI_lib_State_Machine.vi"("State(s) in (\"\")"=w233) -> ("States Out"=w232:string)  [unwired: 14 in]
      }
      frame "Parameter: Combin Parameter" {
        n104 = property on="方法(Method)" class="Enum (strict)"() -> ("RingText.Text"=w280:string)  [unwired: 2 in, 2 out]
        n105 = Unbundle By Name(w278) -> ("TimeClusters"=w277:T5)
        n106 = case shown="\"Wait_s\"" w280 {
          selector: w280 -> [_ w288 w296 w304]
          tunnel: w277 -> [_ w294 w302 w310]
          tunnel: [_ w292 w300 w308] -> w279
          tunnel: [w286 w287 w295 w303] -> w282
          tunnel: w281 -> [w286 w290 w298 w306]
          frame Default {
          }
          frame "Wait_ms" {
            n107 = Unbundle By Name(w294) -> ("Initialize"=w293:T11)
            n108 = Bundle By Name(cluster=w293, "json.Method"=w288) -> (w289:T11)
            n109 = call <vilib>:"Flatten To JSON String.vi"("Multiline (T)"=TRUE, "error in (no error)"=w290, "Variant"=w289) -> ("error out"=w287:errorcluster, "JSON String"=w292:string)  [unwired: 7 in]
          }
          frame "Wait_s" {
            n110 = Unbundle By Name(w302) -> ("SetVoltage"=w301:T12)
            n111 = Bundle By Name(cluster=w301, "json.Method"=w296) -> (w297:T12)
            n112 = call <vilib>:"Flatten To JSON String.vi"("Multiline (T)"=TRUE, "error in (no error)"=w298, "Variant"=w297) -> ("error out"=w295:errorcluster, "JSON String"=w300:string)  [unwired: 7 in]
          }
          frame "TickCount" {
            n113 = Unbundle By Name(w310) -> ("SetCurrent"=w309:cluster{"json":cluster{"Method":string}})
            n114 = Bundle By Name(cluster=w309, "json.Method"=w304) -> (w305:cluster{"json":cluster{"Method":string}})
            n115 = call <vilib>:"Flatten To JSON String.vi"("Multiline (T)"=TRUE, "error in (no error)"=w306, "Variant"=w305) -> ("error out"=w303:errorcluster, "JSON String"=w308:string)  [unwired: 7 in]
          }
        }
        n116 = Bundle By Name(cluster=w278, "Synchronize.Echo.JsonOut"=w279) -> (w283:T8)
        n117 = call <vilib>:"Add State(s) to Queue__JKI_lib_State_Machine.vi"("State(s) in (\"\")"=w285) -> ("States Out"=w284:string)  [unwired: 14 in]
      }
      frame "---------- Sync ----------" {
        n118 = call <vilib>:"Add State(s) to Queue__JKI_lib_State_Machine.vi"("State(s) in (\"\")"=w314) -> ("States Out"=w313:string)  [unwired: 14 in]
      }
      frame "Sync: Obtain CMD Queue" {
        # "这里由平台输入"
        n119 = Unbundle By Name(w316) -> ("Synchronize.EnqueueData"=w315:T13)
        n120 = Obtain Queue(name (unnamed)="VIId", element data type=w315, error in (no error)=w321) -> (queue out=w317:refnum<queue>, error out=w320:errorcluster)  [unwired: 2 in, 1 out]
        n121 = Bundle By Name(cluster=w316, "Synchronize.Queue"=w317) -> (w318:T8)
        n122 = call <vilib>:"Add State(s) to Queue__JKI_lib_State_Machine.vi"("State(s) in (\"\")"=w323) -> ("States Out"=w322:string)  [unwired: 14 in]
      }
      frame "Sync: Dequeue CMD" {
        n123 = Unbundle By Name(w336) -> ("Synchronize.Queue"=w333:refnum<queue>, "Synchronize.Communicate"=w324:T14)
        n124 = Dequeue Element(queue=w333, timeout in ms (-1)=10, error in (no error)=w334) -> (queue out=w332:refnum<queue>, element=w330:T13, timed out?=w331:bool, error out=w326:errorcluster)
        n125 = Bundle By Name(cluster=w336, "Synchronize.Queue"=w332, "Synchronize.EnqueueData"=w330) -> (w328:T8)
        n126 = case shown="False" w331 {
          tunnel: w330 -> [w347 _]
          tunnel: [w345 _] -> w329
          tunnel: w328 -> [w344 w376]
          tunnel: [w343 w376] -> w327
          tunnel: w326 -> [w341 w375]
          tunnel: [w340 w375] -> w325
          tunnel: w324 -> [w339 _]
          frame False {
            n127 = Unbundle By Name(w347) -> ("Action"=w346:T15, "Data"=w342:variant)
            n128 = case shown="\"Query\"" w346 {
              tunnel: ["Sync: Send ECHO" "UI: Initialize VarList\nSync: Send ECHO" _ "Sync: Send ECHO\nMacro: Exit" "Parameter: Combin Parameter\nSync: Send ECHO" "Parameter: Parse Parameter\nSync: Send ECHO"] -> w345
              tunnel: w344 -> [w350 w355 w359 w362 w367 w372]
              tunnel: [w349 w354 w359 w361 w366 w371] -> w343
              tunnel: w342 -> [_ _ _ _ _ _]
              tunnel: w341 -> [w351 w356 w358 w363 w368 w373]
              tunnel: [w351 w356 w358 w363 w368 w373] -> w340
              tunnel: w339 -> [_ _ _ _ _ _]
              frame "Create" {
                n129 = Bundle By Name(cluster=w350, "Synchronize.Echo.Status"="Create Success") -> (w349:T8)
              }
              frame "UpdateVariable" {
                n130 = Bundle By Name(cluster=w355, "Synchronize.Echo.Status"="UpdateVariable Success") -> (w354:T8)
              }
              frame Default {
              }
              frame "Close" {
                n131 = Bundle By Name(cluster=w362, "Synchronize.Echo.Status"="Close Success") -> (w361:T8)
              }
              frame "Query" {
                n132 = Bundle By Name(cluster=w367, "Synchronize.Echo.Status"="Query Success") -> (w366:T8)
              }
              frame "Revert" {
                n133 = Bundle By Name(cluster=w372, "Synchronize.Echo.Status"="Revert Success") -> (w371:T8)
              }
            }
          }
          frame True {
          }
        }
        n134 = call <vilib>:"Add State(s) to Queue__JKI_lib_State_Machine.vi"("State(s) in Front (\"\")"=w329, "State(s) in (\"\")"=w338) -> ("States Out"=w337:string)  [unwired: 13 in]
      }
      frame "Sync: Release CMD Queue" {
        n135 = Unbundle By Name(w379) -> ("Synchronize.Queue"=w380:refnum<queue>)
        n136 = Release Queue(queue=w380, error in (no error)=w378) -> (error out=w377:errorcluster)  [unwired: 1 in, 2 out]
        n137 = call <vilib>:"Add State(s) to Queue__JKI_lib_State_Machine.vi"("State(s) in (\"\")"=w382) -> ("States Out"=w381:string)  [unwired: 14 in]
      }
      frame "Sync: Send ECHO" {
        n138 = Unbundle By Name(w386) -> ("Synchronize.Communicate"=w383:T14, "Synchronize.EnqueueData.Data"=w395:variant, "Synchronize.Echo"=w387:T16)
        n139 = Variant To Data(error in=w385, type=w383, Variant=w395) -> (data=w388:T14, error out=w389:errorcluster)
        n140 = Unbundle By Name(w388) -> ("ID"=w392:string)
        n141 = Obtain Queue(name (unnamed)=w392, element data type=w387, error in (no error)=w389) -> (queue out=w391:refnum<queue>, error out=w393:errorcluster)  [unwired: 2 in, 1 out]
        n142 = Enqueue Element(queue=w391, element=w387, error in (no error)=w393) -> (queue out=w390:refnum<queue>, error out=w394:errorcluster)  [unwired: 1 in, 1 out]
        n143 = Release Queue(queue=w390, error in (no error)=w394) -> (error out=w384:errorcluster)  [unwired: 1 in, 2 out]
        n144 = call <vilib>:"Add State(s) to Queue__JKI_lib_State_Machine.vi"("State(s) in (\"\")"=w397) -> ("States Out"=w396:string)  [unwired: 14 in]
      }
    }
  }
  n145 = flat-sequence {
    frame #0 {
    }
  }
